vi "Acquire.vi"(8 "error in (no error)":errorcluster, 11 "Refnum in":refnum<k21>) -> (0 "error out":errorcluster, 2 "Graph Data":waveform(dbl)[](array[waveform]))   [LabVIEW 2019, in "Acquisition.lvlib"]
doc: "Perform the acquisition. Replace the contents of this diagram with calls to acquisition hardware.\n_____\nBased on Delacor QMH Project Template 5.0.0.82."
uses:
  Acquisition.lvlib
  <vilib>/ULx/Create Channel.llb/ULx Create Channel (AI-Temperature).vi
  <vilib>/ULx/Read.llb/ULx Read (Analog DBL 1Chan 1Samp).vi
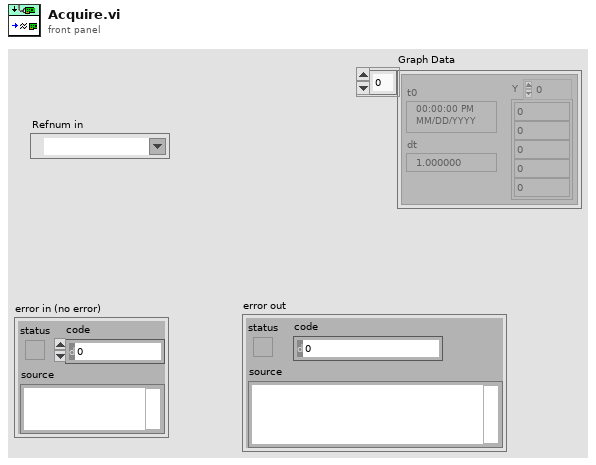
[diagram p1: front panel]
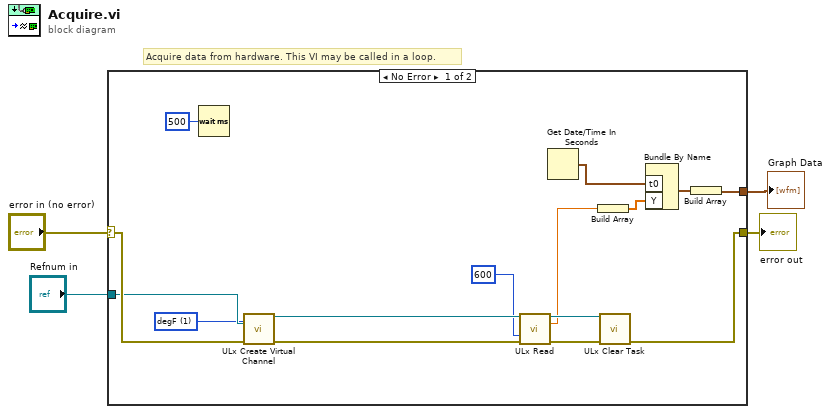
[diagram p0: block diagram]
diagram:
  # "Acquire data from hardware. This VI may be called in a loop."
  n1 = case shown="No Error" "error in (no error)" {
    selector: "error in (no error)" -> [w13 w20]
    tunnel: [w14 w20] -> w3
    tunnel: [w11 _] -> w2
    tunnel: "Refnum in" -> [w12 _]
    frame No Error {
      w10 = 1 items=["degC", "degF", "kelvin", "raw"] ("units")
      n2 = Wait (ms)(milliseconds to wait=u32 500) -> ()  [unwired: 1 out]
      n3 = call-poly <vilib>:"ULx Create Virtual Channel.vi"("physical channels"=w12, "units"=w10, "error in"=w13) -> ("task out"=w18:refnum<k24>, "error out"=w19:errorcluster)  [unwired: 11 in]
      n4 = call-poly <vilib>:"ULx Read.vi"("task in"=w18, "timeout"=600, "error in"=w19) -> ("task out"=w17:refnum<k24>, "data"=w8:dbl, "error out"=w16:errorcluster)  [unwired: 10 in]
      n5 = Get Date/Time In Seconds() -> (seconds since 1Jan1904=w9:timestamp)
      n6 = Build Array(w8) -> (w7:dbl[])
      n7 = call <vilib>:"ULx Clear Task.vi"("task in"=w17, "error in"=w16) -> ("error out"=w14:errorcluster)  [unwired: 13 in]
      n8 = Bundle By Name("t0"=w9, "Y"=w7) -> (w6:waveform(dbl))  [unwired: 1 in]
      n9 = Build Array(w6) -> (w11:waveform(dbl)[])
    }
    frame Error {
    }
  }
  "error out" <- w3
  "Graph Data" <- w2
